vi "NXT_master_final.vi"   [LabVIEW 2016]
uses:
  <vilib>/NXT/Block Support/NXT_InputPort.ctl
  <vilib>/NXT/Block Support/HWPage.SensorType.ctl
  <vilib>/NXT/Block Support/HWPage.SensorMode.ctl
  <vilib>/NXT/Block Support/NXT_OutputPort.ctl
  <vilib>/NXT/Dual Mode Library/Sensors/i2c_sensors_big.vi
  <vilib>/NXT/Dual Mode Library/Display/drawText_Right.vi
  <vilib>/NXT/Dual Mode Library/prims/inRangeAndCoerce/inRangeAndCoerce_int8.vi
  <vilib>/NXT/Dual Mode Library/prims/addArrayElements_int.vi
  <vilib>/NXT/NXTIO Xnodes/NXTIONodeSubVIs/NXTMoveMotors.vi
  <vilib>/NXT/Dual Mode Library/Display/drawText.vi
  <vilib>/NXT/Subs/LVHSConnector.ctl
  <vilib>/NXT/NXTIO Xnodes/AddressXNode/NXTIOAddress.xnode
  <vilib>/NXT/NXTIO Xnodes/NXTIOXNode/NXTIO.xnode
  <vilib>/NXT/LegoClasses/BrickReference/BrickReference.lvclass
types:
  T1 = typedef "HWPage.SensorType.ctl" = u8
  T2 = typedef "HWPage.SensorMode.ctl" = u8
  T3 = typedef "NXT_InputPort.ctl" = u32
  T4 = typedef "LVHSConnector.ctl" = refnum<class "BrickReference.lvclass">
  T5 = typedef "NXT_OutputPort.ctl" = u8
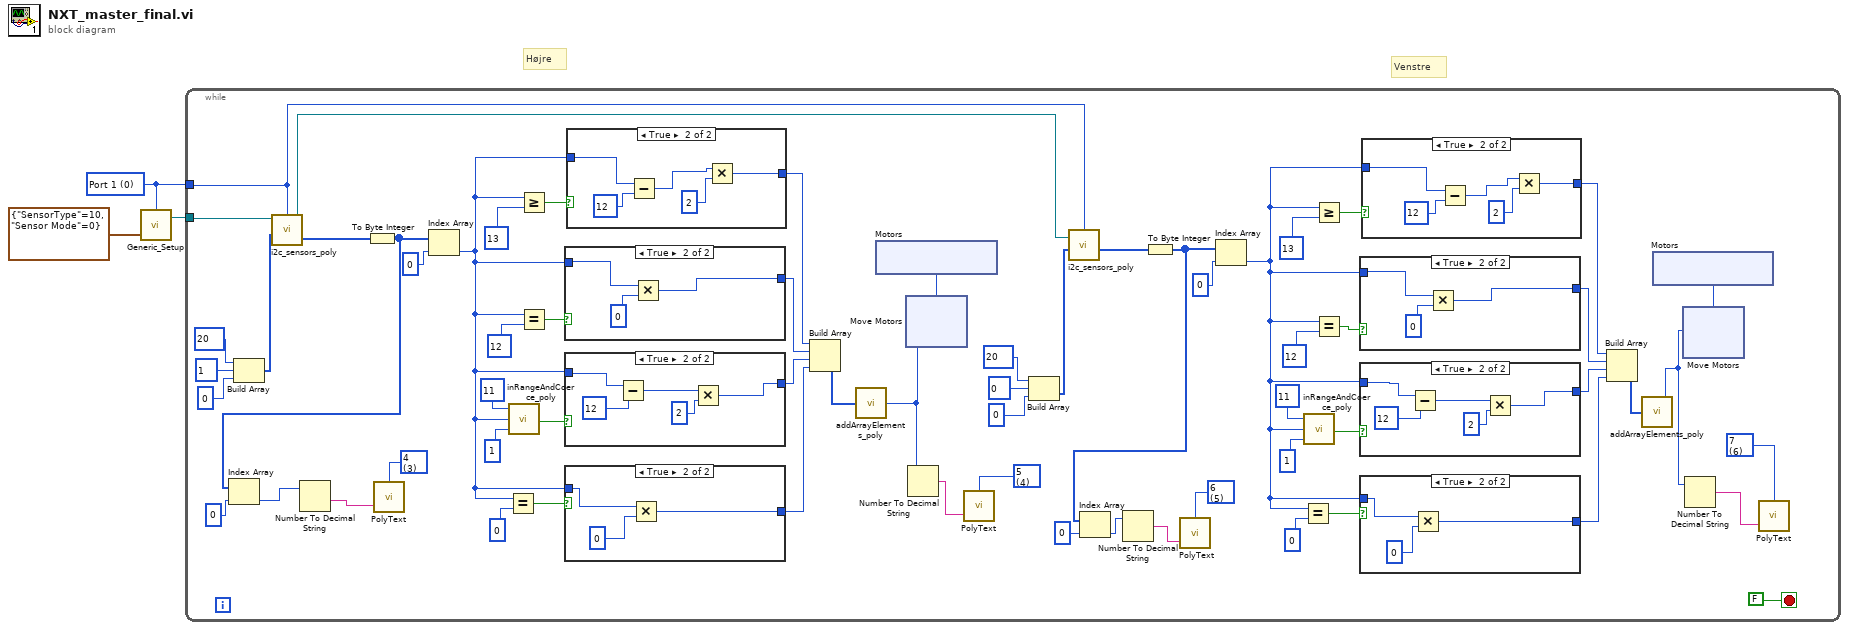
[diagram p0: block diagram]
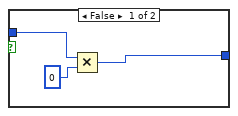
[diagram p2: hidden frame]
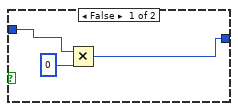
[diagram p3: hidden frame]
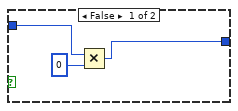
[diagram p4: hidden frame]
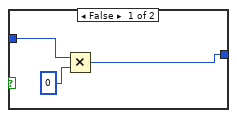
[diagram p5: hidden frame]
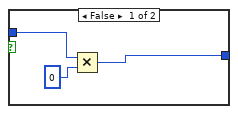
[diagram p6: hidden frame]
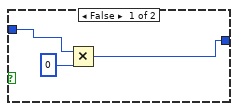
[diagram p7: hidden frame]
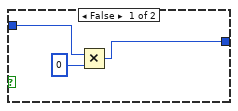
[diagram p8: hidden frame]
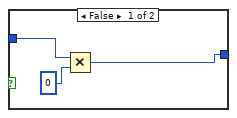
[diagram p9: hidden frame]
diagram:
  w1 = T3 0 items=["Port 1", "Port 2", "Port 3", "Port 4"] ("Port")
  # "Venstre"
  # "Højre"
  n1 = call <vilib>:"Generic_Setup.vi"("Sensor Setup"=cluster{"SensorType":T1, "Sensor Mode":T2} {"SensorType"=10, "Sensor Mode"=0}, "Port"=w1) -> ("NXT/EV3"=w2:T4)  [unwired: 1 in, 1 out]
  n2 = while {
    tunnel: w2 -> [w67]
    tunnel: w1 -> [w66]
    stop <- FALSE stop-if-true
    w6 = i16 6 items=["1", "2", "3", "4", "5", "6", "7", "8", "9", "10", "11", "12"] ("Line")
    w31 = i16 5 items=["1", "2", "3", "4", "5", "6", "7", "8", "9", "10", "11", "12"] ("Line")
    w36 = i16 3 items=["1", "2", "3", "4", "5", "6", "7", "8", "9", "10", "11", "12"] ("Line")
    w40 = i16 4 items=["1", "2", "3", "4", "5", "6", "7", "8", "9", "10", "11", "12"] ("Line")
    n3 = Build Array(u8 20, 1, 0 ("element")) -> (w62:i32[])
    n4 = call-poly <vilib>:"i2c_sensors_poly.vi"("Bytes to Write"=w62, "NXT/EV3"=w67, "Port"=w66) -> ("Bytes read"=w33:u8[], "NXT/EV3"=w56:T4)  [unwired: 2 in, 1 out]
    n5 = To Byte Integer(number=w33) -> (8bit integer=w26:i8[])
    n6 = Index Array(array=w26, index=0) -> (element=w32:i8)
    n7 = Number To Decimal String(number=w32) -> (decimal integer string=w34:string)  [unwired: 1 in]
    n8 = call-poly <vilib>:"PolyText.vi"("Text"=w34, "Line"=w36) -> ()  [unwired: 2 in, 1 out]
    n9 = Index Array(array=w26, index=0) -> (element=w37:i8)
    n10 = Equal?(x=w37, y=i8 0) -> (x = y?=w48:bool)
    n11 = call-poly <vilib>:"inRangeAndCoerce_poly.vi"("lower limit"=i8 1, "x"=w37, "upper limit"=i8 11) -> ("In Range?"=w52:bool)  [unwired: 1 out]
    n12 = Greater Or Equal?(x=w37, y=i8 13) -> (x >= y?=w44:bool)
    n13 = Equal?(x=w37, y=i8 12) -> (x = y?=w46:bool)
    n14 = case shown="True" w46 {
      tunnel: w37 -> [w119 w122]
      tunnel: [w118 w121] -> w42
      frame False {
        n15 = Multiply(x=w119, y=i8 0) -> (x*y=w118:i8)
      }
      frame True {
        n16 = Multiply(x=w122, y=i8 0) -> (x*y=w121:i8)
      }
    }
    n17 = case shown="True" w52 {
      tunnel: w37 -> [w111 w116]
      tunnel: [w110 w113] -> w41
      frame False {
        n18 = Multiply(x=w111, y=i8 0) -> (x*y=w110:i8)
      }
      frame True {
        n19 = Subtract(x=w116, y=i8 12) -> (x-y=w117:i8)
        n20 = Multiply(x=w117, y=i8 2) -> (x*y=w113:i8)
      }
    }
    n21 = case shown="True" w48 {
      tunnel: w37 -> [w105 w108]
      tunnel: [w104 w107] -> w38
      frame False {
        n22 = Multiply(x=w105, y=i8 0) -> (x*y=w104:i8)
      }
      frame True {
        n23 = Multiply(x=w108, y=i8 0) -> (x*y=w107:i8)
      }
    }
    n24 = case shown="True" w44 {
      tunnel: [w124 w130] -> w43
      tunnel: w37 -> [w125 w129]
      frame False {
        n25 = Multiply(x=w125, y=i8 0) -> (x*y=w124:i8)
      }
      frame True {
        n26 = Subtract(x=w129, y=i8 12) -> (x-y=w127:i8)
        n27 = Multiply(x=w127, y=i8 2) -> (x*y=w130:i8)
      }
    }
    n28 = Build Array "Build Array"(w43, w42, w41, w38) -> (w5:i8[])
    n29 = call-poly <vilib>:"addArrayElements_poly.vi"("Numeric Array"=w5) -> ("Sum"=w4:i32)
    n30 = xnode "Motors"() -> ("Motor"=w57:T5)
    n31 = xnode "Move Motors"("Power/Speed 1"=w4, "Motors"=w57) -> ()  [unwired: 1 in, 1 out]
    n32 = Number To Decimal String(number=w4) -> (decimal integer string=w39:string)  [unwired: 1 in]
    n33 = call-poly <vilib>:"PolyText.vi"("Text"=w39, "Line"=w40) -> ()  [unwired: 2 in, 1 out]
    n34 = Build Array(u8 20, 0, 0 ("element")) -> (w58:i32[])
    n35 = call-poly <vilib>:"i2c_sensors_poly.vi"("Bytes to Write"=w58, "NXT/EV3"=w56, "Port"=w66) -> ("Bytes read"=w27:u8[])  [unwired: 2 in, 2 out]
    n36 = To Byte Integer(number=w27) -> (8bit integer=w25:i8[])
    n37 = Index Array(array=w25, index=0) -> (element=w28:i8)
    n38 = Number To Decimal String(number=w28) -> (decimal integer string=w29:string)  [unwired: 1 in]
    n39 = call-poly <vilib>:"PolyText.vi"("Text"=w29, "Line"=w31) -> ()  [unwired: 2 in, 1 out]
    n40 = Index Array(array=w25, index=0) -> (element=w7:i8)
    n41 = Equal?(x=w7, y=i8 0) -> (x = y?=w19:bool)
    n42 = call-poly <vilib>:"inRangeAndCoerce_poly.vi"("lower limit"=i8 1, "x"=w7, "upper limit"=i8 11) -> ("In Range?"=w23:bool)  [unwired: 1 out]
    n43 = Greater Or Equal?(x=w7, y=i8 13) -> (x >= y?=w15:bool)
    n44 = Equal?(x=w7, y=i8 12) -> (x = y?=w17:bool)
    n45 = case shown="True" w17 {
      tunnel: w7 -> [w83 w86]
      tunnel: [w82 w85] -> w12
      frame False {
        n46 = Multiply(x=w83, y=i8 0) -> (x*y=w82:i8)
      }
      frame True {
        n47 = Multiply(x=w86, y=i8 0) -> (x*y=w85:i8)
      }
    }
    n48 = case shown="True" w23 {
      tunnel: w7 -> [w75 w77]
      tunnel: [w74 w78] -> w11
      frame False {
        n49 = Multiply(x=w75, y=i8 0) -> (x*y=w74:i8)
      }
      frame True {
        n50 = Subtract(x=w77, y=i8 12) -> (x-y=w81:i8)
        n51 = Multiply(x=w81, y=i8 2) -> (x*y=w78:i8)
      }
    }
    n52 = case shown="True" w19 {
      tunnel: w7 -> [w69 w72]
      tunnel: [w68 w71] -> w8
      frame False {
        n53 = Multiply(x=w69, y=i8 0) -> (x*y=w68:i8)
      }
      frame True {
        n54 = Multiply(x=w72, y=i8 0) -> (x*y=w71:i8)
      }
    }
    n55 = case shown="True" w15 {
      tunnel: [w88 w94] -> w14
      tunnel: w7 -> [w89 w93]
      frame False {
        n56 = Multiply(x=w89, y=i8 0) -> (x*y=w88:i8)
      }
      frame True {
        n57 = Subtract(x=w93, y=i8 12) -> (x-y=w91:i8)
        n58 = Multiply(x=w91, y=i8 2) -> (x*y=w94:i8)
      }
    }
    n59 = Build Array(w14, w12, w11, w8) -> (w13:i8[])
    n60 = call-poly <vilib>:"addArrayElements_poly.vi"("Numeric Array"=w13) -> ("Sum"=w9:i32)
    n61 = xnode "Motors"() -> ("Motor"=w24:T5)
    n62 = xnode "Move Motors"("Power/Speed 1"=w9, "Motors"=w24) -> ()  [unwired: 1 in, 1 out]
    n63 = Number To Decimal String(number=w9) -> (decimal integer string=w10:string)  [unwired: 1 in]
    n64 = call-poly <vilib>:"PolyText.vi"("Text"=w10, "Line"=w6) -> ()  [unwired: 2 in, 1 out]
  }
